vi "Move.vi"(8 "error in (no error)":errorcluster, 11 "PongBall in":refnum<class "PongBall.lvclass">) -> (0 "error out":errorcluster, 3 "PongBall out":refnum<class "PongBall.lvclass">)   [LabVIEW 2019, in "RT_Game.lvlib" / "PongBall.lvclass"]
uses:
  PongBall.lvclass
  C:/Users/FreshBob/Dropbox/VIs/myRIO_GameConsole/RT/RT_Game/GameObject/GameObject.lvclass
  GameObject/GameObject.lvclass/GameObject.ctl
  GameObject/Read position.vi
  GameObject/Read Velocity.vi
  GameObject/Read Gravity.vi
  GameObject/Write position.vi
  GameObject/Write Velocity.vi
  Globals.vi
  RT_Game.lvlib
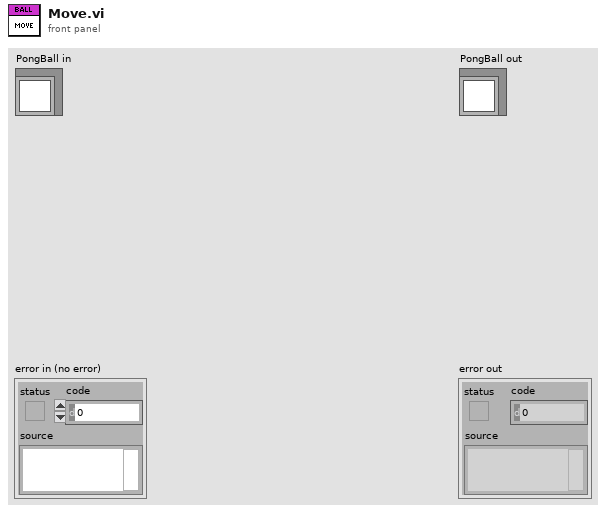
[diagram p1: front panel]
types:
  T1 = typedef "RT_Game.lvlib/Game.lvclass/Coordinate.ctl" = cluster{"x":dbl, "y":dbl}
  T2 = typedef "Velocity.ctl" = cluster{"x":dbl, "y":dbl}
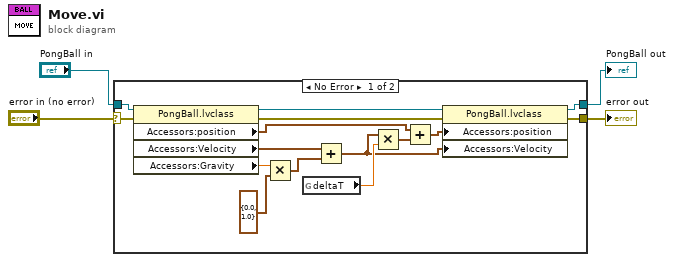
[diagram p0: block diagram]
diagram:
  n1 = case shown="No Error" "error in (no error)" {
    selector: "error in (no error)" -> [w15 w21]
    tunnel: [w16 w21] -> w3
    tunnel: [w19 w20] -> w1
    tunnel: "PongBall in" -> [w12 w20]
    frame No Error {
      n2 = property class="PongBall.lvclass"(reference=w12, error in=w15) -> (reference out=w18:refnum<class "PongBall.lvclass">, error out=w17:errorcluster, "Accessors:position"=w14:T1, "Accessors:Velocity"=w9:T2, "Accessors:Gravity"=w5:dbl)
      n3 = Multiply(x=w5, y=cluster{"x":dbl, "y":dbl} {"x"=0.0, "y"=1.0} ("x")) -> (x*y=w6:cluster{"x":dbl, "y":dbl})
      n4 = global read "Globals.vi" "deltaT"() -> (w10:dbl)
      n5 = Add(x=w9, y=w6) -> (x+y=w8:T2)
      n6 = Multiply(x=w8, y=w10) -> (x*y=w11:T2)
      n7 = Add(x=w14, y=w11) -> (x+y=w13:T1)
      n8 = property class="PongBall.lvclass"(reference=w18, error in=w17, "Accessors:position"=w13, "Accessors:Velocity"=w8) -> (reference out=w19:refnum<class "PongBall.lvclass">, error out=w16:errorcluster)
    }
    frame Error {
    }
  }
  "error out" <- w3
  "PongBall out" <- w1
